vi "Get Bitfile Version.vi"(8 "error in (no error)":errorcluster, 11 "Item Ref in":T2 format="%.0x") -> (0 "error out":errorcluster, 2 "EST version enum":T1, 3 "Item Ref out":T2 format="%.0x", 4 "valid":bool)   [LabVIEW 2013, in "Engine Simulation Toolkit System Explorer.lvlib"]
uses:
  Engine Simulation Toolkit System Explorer.lvlib
  <vilib>/NI Veristand/Custom Device API/Custom Device Item Ref.ctl
  Shared/Bitfile EST Version.ctl
  <vilib>/NI Veristand/Custom Device Tools/Custom Device Utility Library/Search Direction.ctl
  Shared/Constants and GUIDs.vi
  <vilib>/NI Veristand/Custom Device Tools/Custom Device Utility Library/NI VeriStand - Search for Item by GUID.vi
  Shared/Properties.vi
  <vilib>/NI Veristand/Custom Device API/Get Item Property (String).vi
  <vilib>/NI Veristand/Custom Device Tools/Custom Device Utility Library/Custom Device Utility Library.lvlib
  Shared/Engine Simulation Toolkit Shared.lvlib
  <vilib>/NI Veristand/Custom Device API/Custom Device API.lvlib
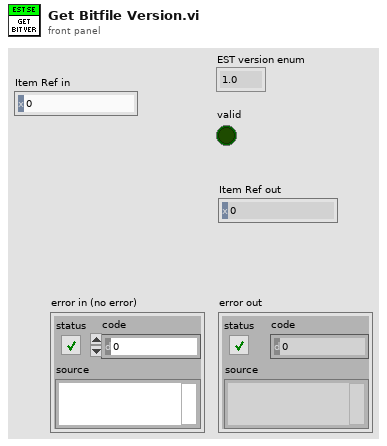
[diagram p1: front panel]
types:
  T1 = typedef "Engine Simulation Toolkit Shared.lvlib/Bitfile EST Version.ctl" = enum16{"1.0", "1.1", "1.2", "1.3"}
  T2 = typedef "Custom Device API.lvlib/Custom Device Item Ref.ctl" = u64
  T3 = typedef "Custom Device Utility Library.lvlib/Search Direction.ctl" = enum16{"Down", "Up"}
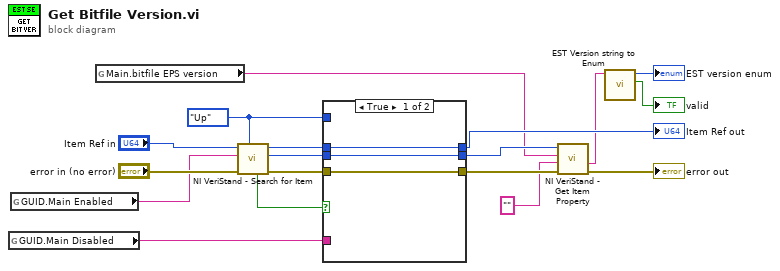
[diagram p0: block diagram]
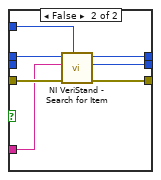
[diagram p2: hidden frame]
diagram:
  w9 = Search_Direction."Up" ("Direction (Down)")
  n1 = global read "Constants and GUIDs.vi" "GUID.Main Disabled"() -> (w10:string)
  n2 = global read "Constants and GUIDs.vi" "GUID.Main Enabled"() -> (w16:string)
  n3 = global read "Properties.vi" "Main.bitfile EPS version"() -> (w5:string)
  n4 = call-poly <vilib>:"NI VeriStand - Search for Item.vi"("Direction (Down)"=w9, "error in"="error in (no error)", "Item GUID"=w16, "Section Ref in"="Item Ref in") -> ("error out"=w13:errorcluster, "Item Ref"=w11:T2, "Section Ref out"=w12:T2, "Found"=w14:bool)  [unwired: 4 in]
  n5 = case shown="True" w14 {
    tunnel: w13 -> [w21 w28]
    tunnel: w12 -> [w19 w27]
    tunnel: w11 -> [w20 _]
    tunnel: w10 -> [_ w26]
    tunnel: w9 -> [_ w25]
    tunnel: [w20 w24] -> w8
    tunnel: [w19 w23] -> w7
    tunnel: [w21 w22] -> w6
    frame True {
    }
    frame False {
      n6 = call-poly <vilib>:"NI VeriStand - Search for Item.vi"("Direction (Down)"=w25, "error in"=w28, "Item GUID"=w26, "Section Ref in"=w27) -> ("error out"=w22:errorcluster, "Item Ref"=w24:T2, "Section Ref out"=w23:T2)  [unwired: 4 in, 1 out]
    }
  }
  "Item Ref out" <- w7
  n7 = call-poly <vilib>:"NI VeriStand - Get Item Property.vi"("error in (no error)"=w6, "Default Value"="", "Property Name"=w5, "Item Ref in"=w8) -> ("error out"=→"error out":errorcluster, "Value"=w3:string)  [unwired: 4 in, 2 out]
  n8 = call "EST Version string to Enum.vi"("EST version string"=w3) -> ("valid"=→"valid":bool, "EST version enum"=→"EST version enum":T1)  [unwired: 9 in]
